vi "Viavi - Build Cell.vi"(0 "Input Value":dbl, 2 "Parameter Input":T1={"Warning High"=inf, "Warning Low"=-inf, "Fail High"=inf, "Fail Low"=-inf, "Display Precision"=0}) -> (7 "Single Cell Cluster":T2)   [LabVIEW 2017]
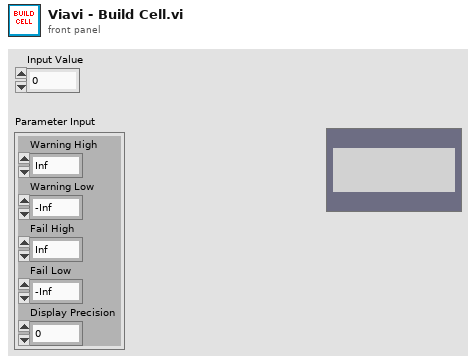
[diagram p1: front panel]
types:
  T1 = cluster{"Warning High":dbl, "Warning Low":dbl, "Fail High":dbl, "Fail Low":dbl, "Display Precision":i32}
  T2 = cluster{"String":string, "Warning":bool, "Fail":bool, "Numeric":dbl}
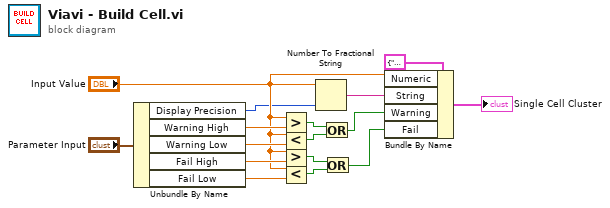
[diagram p0: block diagram]
diagram:
  n1 = Unbundle By Name("Parameter Input") -> ("Display Precision"=w1:i32, "Warning High"=w14:dbl, "Warning Low"=w13:dbl, "Fail High"=w12:dbl, "Fail Low"=w11:dbl)
  n2 = Greater?(x="Input Value", y=w14) -> (0:w10:bool)
  n3 = Less?(x="Input Value", y=w13) -> (x < y?=w9:bool)
  n4 = Greater?(x="Input Value", y=w12) -> (0:w8:bool)
  n5 = Less?(x="Input Value", y=w11) -> (x < y?=w7:bool)
  n6 = Number To Fractional String(number="Input Value", precision (6)=w1) -> (F-format string=w16:string)  [unwired: 2 in]
  n7 = Or(x=w10, y=w9) -> (x .or. y?=w5:bool)
  n8 = Or(x=w8, y=w7) -> (x .or. y?=w6:bool)
  n9 = Bundle By Name(cluster=T2 {"String"="", "Warning"=TRUE, "Fail"=TRUE, "Numeric"=0.0} ("Single Cell Cluster"), "Numeric"="Input Value", "String"=w16, "Warning"=w5, "Fail"=w6) -> (→"Single Cell Cluster":T2)
